vi "Spectrometer iHR320.vi"(8 "error in (no error)":errorcluster, 11 "Spect. iHR320 In":refnum<class "Spectrometer iHR320.lvclass">) -> (0 "error out":errorcluster, 3 "Spectr. iHR320 Out":refnum<class "Spectrometer iHR320.lvclass">)   [LabVIEW 2009, in "Spectrometer iHR320.lvclass"]
doc: "Creates the iHR 320 Spectrometer object.\n\nCan also control the TRIAX 550 if the Unique ID is set to Mono1 instead of Mono2."
uses:
  Spectrometer iHR320.lvclass
  Global/GPIB Numbers.vi
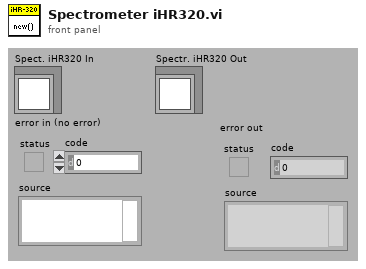
[diagram p1: front panel]
types:
  T1 = typedef "USBMono Type Def.ctl" = cluster{"Name":string, "Unique ID":string}
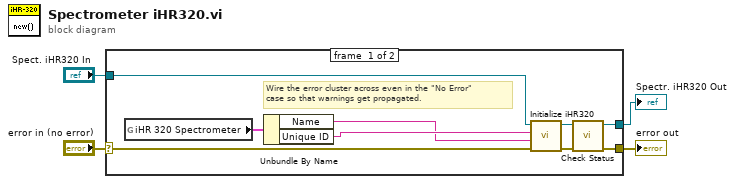
[diagram p0: block diagram]
diagram:
  n1 = case shown="No Error" "error in (no error)" {
    selector: "error in (no error)" -> [w11 w15]
    tunnel: [w7 w15] -> w2
    tunnel: [w9 w14] -> w3
    tunnel: "Spect. iHR320 In" -> [w12 w14]
    frame #0 {
      # "Wire the error cluster across even in the \"No Error\"\ncase so that warnings get propagated."
      n2 = global read "GPIB Numbers.vi" "iHR 320 Spectrometer"() -> (w13:T1)
      n3 = Unbundle By Name(w13) -> ("Name"=w5:string, "Unique ID"=w6:string)
      n4 = call "Initialize iHR320.vi"("error in (no error)"=w11, "Mono ID"=w5, "Unique ID"=w6, "Spectrometer iHR320 In"=w12) -> ("error out"=w8:errorcluster, "Spectrometer iHR320 Out"=w10:refnum<class "Spectrometer iHR320.lvclass">)  [unwired: 5 in, 1 out]
      n5 = call-dynamic "Check Status.vi"("error in (no error)"=w8, "Spectrometer iHR320 in"=w10) -> ("error out"=w7:errorcluster, "Spectrometer iHR320 out"=w9:refnum<class "Spectrometer iHR320.lvclass">)  [unwired: 6 in, 2 out]
    }
    frame #1 {
    }
  }
  "error out" <- w2
  "Spectr. iHR320 Out" <- w3
